vi "Count coincidence multiplicity.vi"(8 "error in":errorcluster, 11 "CRT-wide coincidences":cluster{"CRT-wide coincs":T1[]}[](array[cluster])) -> (0 "error out":errorcluster, 3 "New data?":bool)   [LabVIEW 2016]
uses:
  Typedefs/Coincidence.ctl
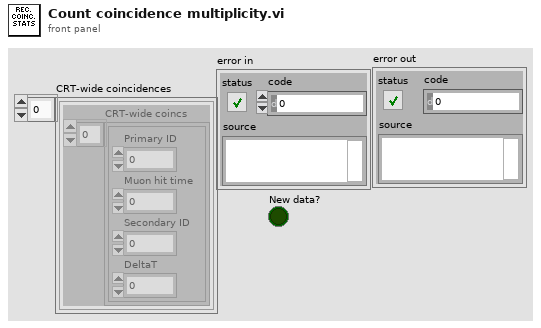
[diagram p1: front panel]
types:
  T1 = typedef "Coincidence.ctl" = cluster{"Primary ID":i8, "Muon hit time":u64, "Secondary ID":i8, "DeltaT":i32}
  T2 = cluster{"Numofpoints":i32, "Current index":i32, "Max index":i32, "Data":cluster{"initialized array":i32[][], "Timestamp":timestamp}[], "Filled":bool}
  T3 = cluster{"initialized array":i32[][], "Timestamp":timestamp}[]
  T4 = cluster{"initialized array":i32[][], "Timestamp":timestamp}
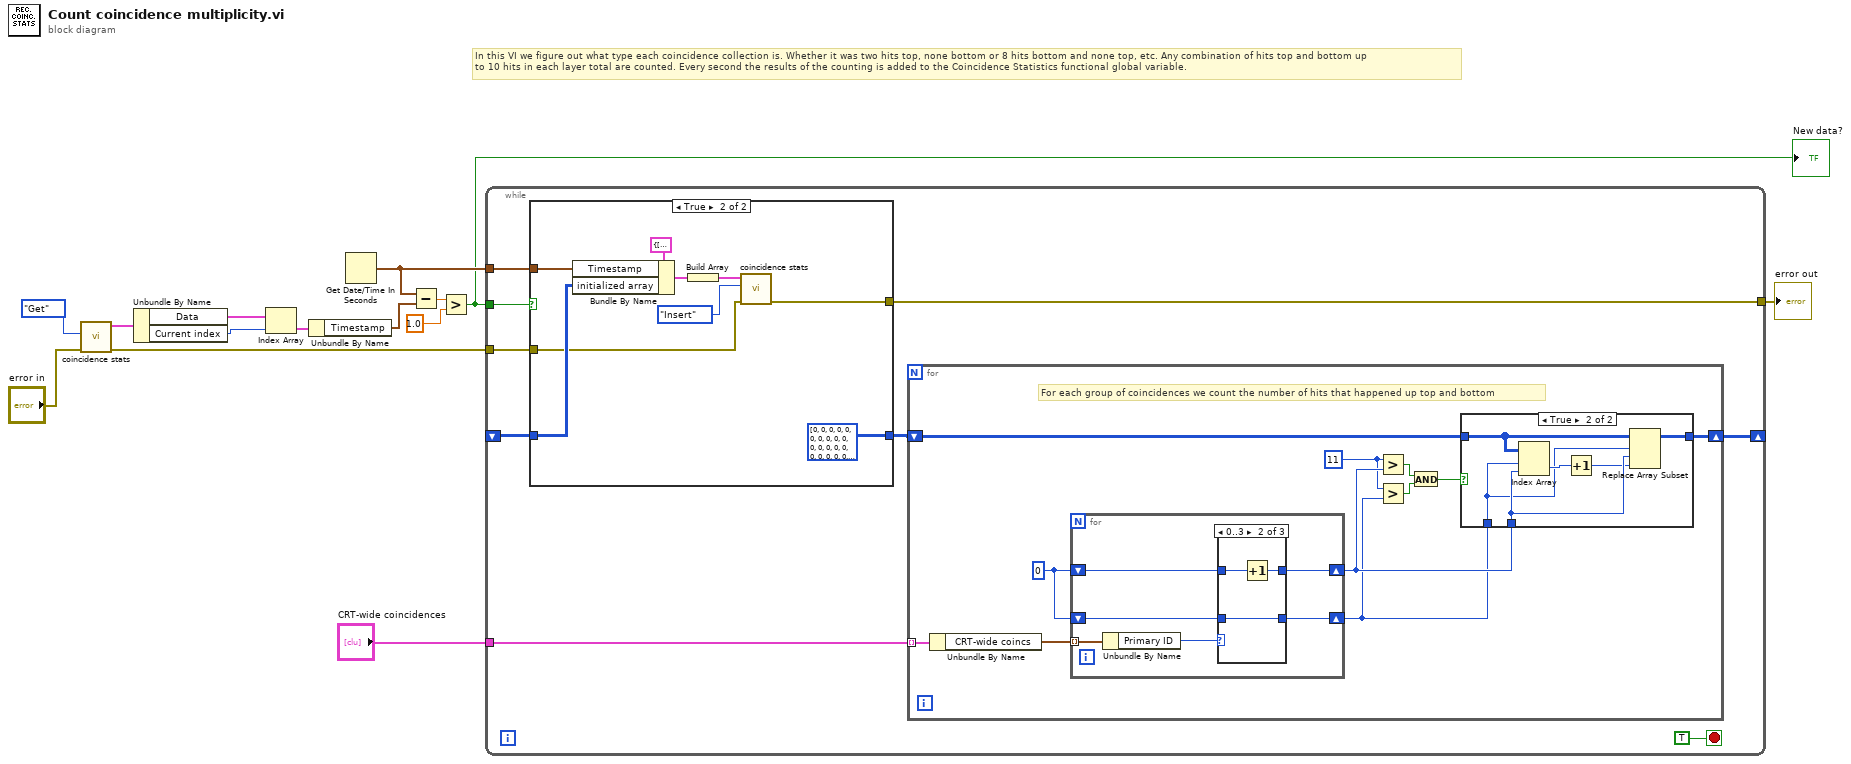
[diagram p0: block diagram]
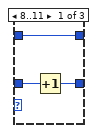
[diagram p4: hidden frame]
diagram:
  # "In this VI we figure out what type each coincidence collection is. Whether it was two hits top, none bottom or 8 hits bottom and none top, etc. Any combination of hits top and bottom up \nto 10 hits in each layer total are counted. Every second the results of the counting is added to the Coincidence Statistics functional global variable."
  n1 = call "coincidence stats.vi"("error in"="error in", "Action"=enum16{"Insert", "Get", "Initiate"}."Get") -> ("error out"=w4:errorcluster, "Coinc stats"=w8:T2)  [unwired: 7 in, 1 out]
  n2 = Unbundle By Name(w8) -> ("Data"=w7:T3, "Current index"=w6:i32)
  n3 = Index Array(array=w7, index=w6) -> (element=w13:T4)
  n4 = Unbundle By Name(w13) -> ("Timestamp"=w12:timestamp)
  n5 = Get Date/Time In Seconds() -> (seconds since 1Jan1904=w5:timestamp)
  n6 = Subtract(x=w5, y=w12) -> (x-y=w11:dbl)
  n7 = Greater?(x=w11, y=1.0) -> (0:w1:bool)
  "New data?" <- w1
  n8 = while {
    tunnel: "CRT-wide coincidences" -> [w23]
    tunnel: w1 -> [w20]
    shift-right: [w18] -> _
    shift-left: _ -> [w19]
    tunnel: w5 -> [w17]
    tunnel: w4 -> [w16]
    tunnel: [w15] -> w2
    stop <- TRUE stop-if-true
    n9 = case shown="True" w20 {
      tunnel: [w25 i32[][] [[0, 0, 0, 0, 0, 0, 0, 0, 0, 0, 0, 0], [0, 0, 0, 0, 0, 0, 0, 0, 0, 0, 0, 0], [0, 0, 0, 0, 0, 0, 0, 0, 0, 0, 0, 0], [0, 0, 0, 0, 0, 0, 0, 0, 0, 0, 0, 0], [0, 0, 0, 0, 0, 0, 0, 0, 0, 0, 0, 0], [0, 0, 0, 0, 0, 0, 0, 0, 0, 0, 0, 0], [0, 0, 0, 0, 0, 0, 0, 0, 0, 0, 0, 0], [0, 0, 0, 0, 0, 0, 0, 0, 0, 0, 0, 0], [0, 0, 0, 0, 0, 0, 0, 0, 0, 0, 0, 0], [0, 0, 0, 0, 0, 0, 0, 0, 0, 0, 0, 0], [0, 0, 0, 0, 0, 0, 0, 0, 0, 0, 0, 0], [0, 0, 0, 0, 0, 0, 0, 0, 0, 0, 0, 0]] ("initialized array")] -> w22
      tunnel: w19 -> [w25 w32]
      tunnel: w17 -> [_ w31]
      tunnel: w16 -> [w24 w27]
      tunnel: [w24 w26] -> w15
      frame False {
      }
      frame True {
        n10 = Bundle By Name(cluster=T4 {"initialized array"=[[0, 0, 0, 0, 0, 0, 0, 0, 0, 0, 0, 0], [0, 0, 0, 0, 0, 0, 0, 0, 0, 0, 0, 0], [0, 0, 0, 0, 0, 0, 0, 0, 0, 0, 0, 0], [0, 0, 0, 0, 0, 0, 0, 0, 0, 0, 0, 0], [0, 0, 0, 0, 0, 0, 0, 0, 0, 0, 0, 0], [0, 0, 0, 0, 0, 0, 0, 0, 0, 0, 0, 0], [0, 0, 0, 0, 0, 0, 0, 0, 0, 0, 0, 0], [0, 0, 0, 0, 0, 0, 0, 0, 0, 0, 0, 0], [0, 0, 0, 0, 0, 0, 0, 0, 0, 0, 0, 0], [0, 0, 0, 0, 0, 0, 0, 0, 0, 0, 0, 0], [0, 0, 0, 0, 0, 0, 0, 0, 0, 0, 0, 0], [0, 0, 0, 0, 0, 0, 0, 0, 0, 0, 0, 0]], "Timestamp"=timestamp(0 s since 1904-01-01)}, "Timestamp"=w31, "initialized array"=w32) -> (w30:T4)
        n11 = Build Array(w30) -> (w29:T3)
        n12 = call "coincidence stats.vi"("error in"=w27, "Action"=enum16{"Insert", "Get", "Initiate"}."Insert", "New data"=w29) -> ("error out"=w26:errorcluster)  [unwired: 6 in, 2 out]
      }
    }
    n13 = for {
      tunnel: w23 -> [w45] mode=indexing
      shift-right: [w41] -> w18
      shift-left: w22 -> [w42]
      w38 = 11 ("x")
      w43 = 0
      # "For each group of coincidences we count the number of hits that happened up top and bottom"
      n14 = Unbundle By Name(w45) -> ("CRT-wide coincs"=w44:T1[])
      n15 = for {
        tunnel: w44 -> [w58] mode=indexing
        shift-right: [w55] -> w40
        shift-left: w43 -> [w56]
        shift-right: [w54] -> w39
        shift-left: w43 -> [w53]
        n16 = Unbundle By Name(w58) -> ("Primary ID"=w57:i8)
        n17 = case shown="0..3" w57 {
          tunnel: w56 -> [w59 w64 w66]
          tunnel: [w59 w63 w66] -> w55
          tunnel: [w60 w62 w65] -> w54
          tunnel: w53 -> [w61 w62 w65]
          frame 8..11 {
            n18 = Increment(x=w61) -> (x+1=w60:i32)
          }
          frame 0..3 {
            n19 = Increment(x=w64) -> (x+1=w63:i32)
          }
          frame Default {
          }
        }
      }
      n20 = Greater?(x=w38, y=w40) -> (0:w36:bool)
      n21 = Greater?(x=w38, y=w39) -> (0:w37:bool)
      n22 = And(x=w36, y=w37) -> (x .and. y?=w35:bool)
      n23 = case shown="True" w35 {
        tunnel: w42 -> [w46 w51]
        tunnel: w40 -> [_ w50]
        tunnel: w39 -> [_ w49]
        tunnel: [w46 w47] -> w41
        frame False {
        }
        frame True {
          n24 = Index Array(array=w51, index (row)=w49, index (col)=w50) -> (element=w52:i32)
          n25 = Increment(x=w52) -> (x+1=w48:i32)
          n26 = Replace Array Subset(array=w51, new element=w48, index (row)=w49, index (col)=w50) -> (w47:i32[][])
        }
      }
    }
  }
  "error out" <- w2
